vi "AlliGator Update Phasor Color Picker Color.vi"(8 "Error In":errorcluster, 9 "New Cursor List in":T1, 11 "XYGraph in":refnum<vi>) -> (0 "Error Out":errorcluster, 1 "New Cursor List out":T1, 2 "Cursor Index":i32, 3 "Cursor Color":u32)   [LabVIEW 2021, in "AlliGator Phasor Plot Color Map.lvlib"]
doc: "Finds out whether the change in the cursor lis tis a color change only. In that case, the calling VI will update the color array accordingly."
uses:
  AlliGator Phasor Plot Color Map.lvlib
  <vilib>/Utility/miscctls.llb/LVCursorListTypeDef.ctl
panel:
  # "see the AlliGator License on the block diagram (Ctrl+E or Window:Show Block Diagram)"
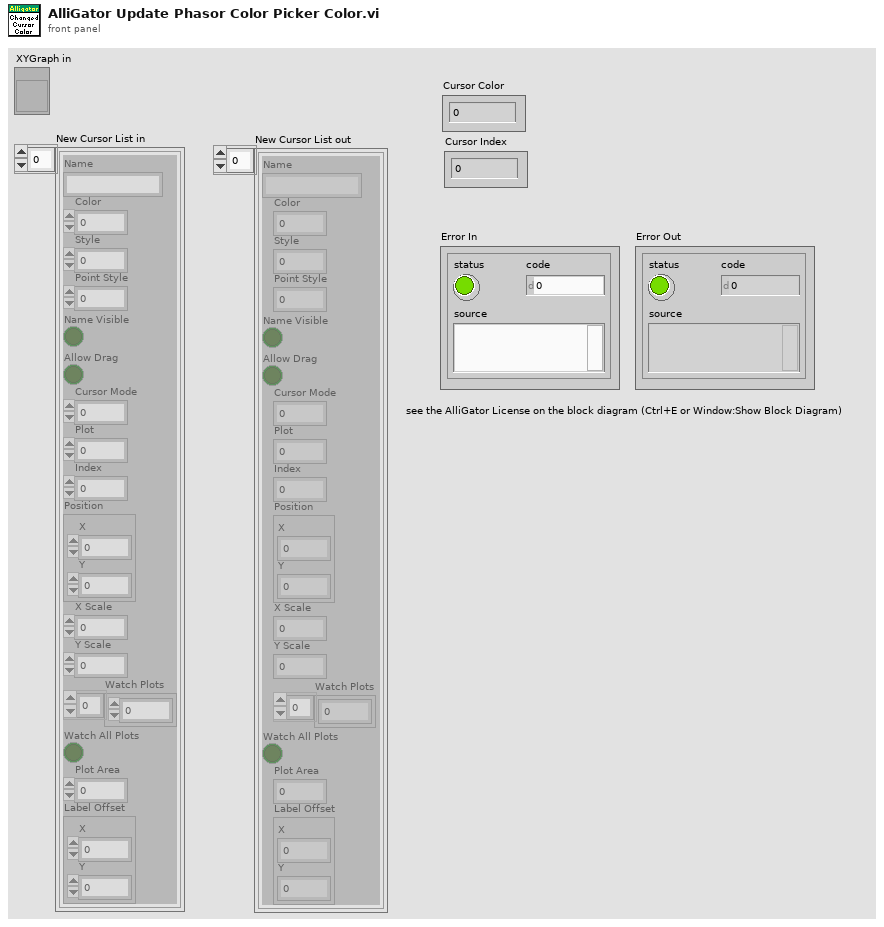
[diagram p1: front panel]
types:
  T1 = typedef "LVCursorListTypeDef.ctl" = cluster{"Name":string, "Color":u32, "Style":u8, "Point Style":u8, "Name Visible":bool, "Allow Drag":bool, "Cursor Mode":u32, "Plot":i32, "Index":i32, "Position":cluster{"X":dbl, "Y":dbl}, "X Scale":u32, "Y Scale":u32, "Watch Plots":i32[], "Watch All Plots":bool, "Plot Area":i32, "Label Offset":cluster{"X":dbl, "Y":dbl}}[]
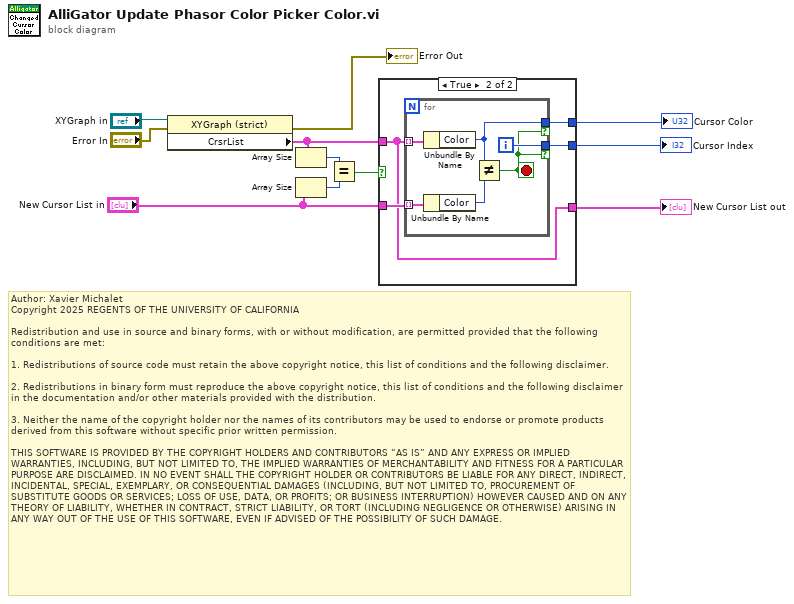
[diagram p0: block diagram]
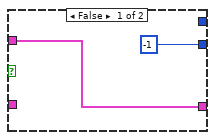
[diagram p2: hidden frame]
diagram:
  # "Author: Xavier Michalet\nCopyright 2025 REGENTS OF THE UNIVERSITY OF CALIFORNIA\n\nRedistribution and use in source and binary forms, with or without modification, are permitted provided that the following conditions are met:\n\n1. Redistributions of source code must retain the above copyright notice, this list of conditions and the following disclaimer.\n\n2. Redistributions in binary form must reproduce the above copyright notice, this list of conditions and the following disclaimer in the documentation and/or other materials provided with the distribution.\n\n3. Neither the name of the copyright holder nor the names of its contributors may be used to endorse or promote products derived from this software without specific prior written permission.\n\nTHIS SOFTWARE IS PROVIDED BY THE COPYRIGHT HOLDERS AND CONTRIBUTORS “AS IS” AND ANY EXPRESS OR IMPLIED WARRANTIES, INCLUDING, BUT NOT LIMITED TO, THE IMPLIED WARRANTIES OF MERCHANTABILITY AND FITNESS FOR A PARTICULAR PURPOSE ARE DISCLAIMED. IN NO EVENT SHALL THE COPYRIGHT HOLDER OR CONTRIBUTORS BE LIABLE FOR ANY DIRECT, INDIRECT, INCIDENTAL, SPECIAL, EXEMPLARY, OR CONSEQUENTIAL DAMAGES (INCLUDING, BUT NOT LIMITED TO, PROCUREMENT OF SUBSTITUTE GOODS OR SERVICES; LOSS OF USE, DATA, OR PROFITS; OR BUSINESS INTERRUPTION) HOWEVER CAUSED AND ON ANY THEORY OF LIABILITY, WHETHER IN CONTRACT, STRICT LIABILITY, OR TORT (INCLUDING NEGLIGENCE OR OTHERWISE) ARISING IN ANY WAY OUT OF THE USE OF THIS SOFTWARE, EVEN IF ADVISED OF THE POSSIBILITY OF SUCH DAMAGE."
  n1 = property class="XYGraph (strict)"(reference="XYGraph in", error in="Error In") -> (error out=→"Error Out":errorcluster, "CrsrList"=w9:T1)  [unwired: 1 out]
  n2 = Array Size(array=w9) -> (size(s)=w7:i32)
  n3 = Array Size(array="New Cursor List in") -> (size(s)=w6:i32)
  n4 = Equal?(x=w7, y=w6) -> (x = y?=w5:bool)
  n5 = case shown="True" w5 {
    tunnel: w9 -> [w13 w14]
    tunnel: "New Cursor List in" -> [_ w17]
    tunnel: [w13 w14] -> w4
    tunnel: [-1 ("Cursor Index") w16] -> w3
    tunnel: [_ w15] -> w2
    frame False {
    }
    frame True {
      n6 = for {
        tunnel: w14 -> [w23] mode=indexing
        tunnel: w17 -> [w22] mode=indexing
        tunnel: [w20] -> w16 if=w18
        tunnel: [w19] -> w15 if=w18
        i -> [w20]
        stop <- w18 stop-if-true
        n7 = Unbundle By Name(w23) -> ("Color"=w19:u32)
        n8 = Unbundle By Name(w22) -> ("Color"=w21:u32)
        n9 = Not Equal?(x=w19, y=w21) -> (x != y?=w18:bool)
      }
    }
  }
  "New Cursor List out" <- w4
  "Cursor Index" <- w3
  "Cursor Color" <- w2
